vi "rm.server.visualize.init.vi"(5 "Splitter":refnum<vi>, 6 "MCLB Reference":refnum<vi>, 7 "menu reference in":refnum<k9>, 8 "error in (no error)":errorcluster, 9 "display":refnum<vi>, 10 "Table Pane in":refnum<vi>, 11 "VI in":refnum<vi>) -> (0 "error out":errorcluster, 2 "selected values":bool[](array[boolean]), 3 "Queue out":refnum<queue>)   [LabVIEW 2016, in "RM.Server.lvlib"]
uses:
  RM.Server.lvlib
  viz_command.ctl
  viz_state.ctl
  Shared/Global Tags.vi
  Shared/RM.Shared.lvlib
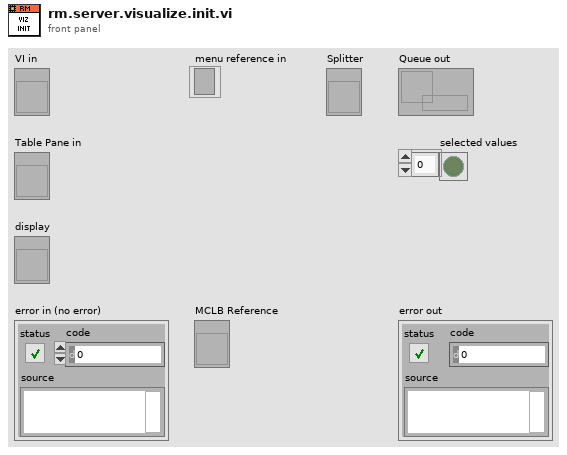
[diagram p1: front panel]
types:
  T1 = enum32{"Invalid", "Standard", "Closed", "Hidden", "Minimized", "Maximized"}
  T2 = typedef "RM.Server.lvlib/viz_command.ctl" = cluster{"state":T3, "data":variant}
  T3 = typedef "RM.Server.lvlib/viz_state.ctl" = enum16{"shutdown"}
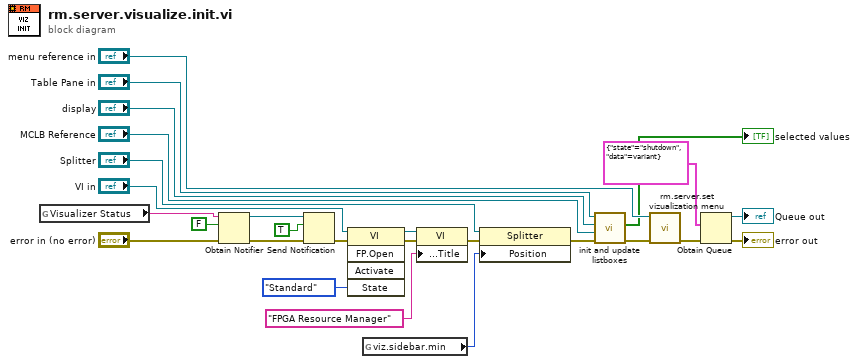
[diagram p0: block diagram]
diagram:
  n1 = global read "Global Tags.vi" "Visualizer Status"() -> (w22:string)
  n2 = Obtain Notifier(name (unnamed)=w22, notification data type=FALSE, error in (no error)="error in (no error)") -> (notifier out=w20:refnum<notifier>, error out=w18:errorcluster)  [unwired: 1 in, 1 out]
  n3 = Send Notification(notification=TRUE, notifier=w20, error in (no error)=w18) -> (error out=w16:errorcluster)  [unwired: 1 out]
  n4 = invoke class="VI" method="FP.Open"(reference="VI in", error in=w16, "State"=T1."Standard") -> (reference out=w11:refnum<vi>, error out=w25:errorcluster)  [unwired: 2 in, 3 out]
  n5 = global read "Global Tags.vi" "viz.sidebar.min"() -> (w7:i32)
  n6 = property class="VI"(reference=w11, error in=w25, "Front Panel.Title"="FPGA Resource Manager" ("Front Panel Window:Title")) -> (error out=w9:errorcluster)  [unwired: 1 out]
  n7 = property on="Property Node" class="Splitter"(reference="Splitter", error in=w9, "Position"=w7) -> (error out=w3:errorcluster)  [unwired: 1 out]
  n8 = call "init and update listboxes.vi"("error in (no error)"=w3, "table"="MCLB Reference", "display"="display", "Pane in"="Table Pane in") -> ("error out"=w2:errorcluster, "selected values"=→"selected values":bool[])  [unwired: 6 in]
  n9 = call "rm.server.set vizualization menu.vi"("error in (no error)"=w2, "menu reference in"="menu reference in") -> ("error out"=w24:errorcluster)  [unwired: 8 in, 1 out]
  n10 = Obtain Queue(element data type=T2 {"state"=enum."shutdown", "data"=variant} ("viz_command"), error in (no error)=w24) -> (queue out=→"Queue out":refnum<queue>, error out=→"error out":errorcluster)  [unwired: 3 in, 1 out]
